vi "mqtt payload to integer.vi"(2 "integer type":i32, 7 "MQTT payload":string="MQTT payload") -> (8 "double":i32, 13 "error out":errorcluster)   [LabVIEW 2017]
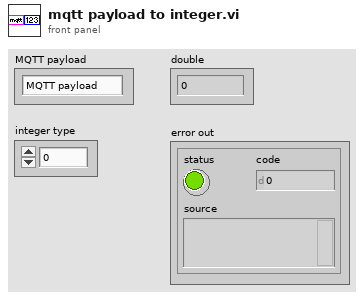
[diagram p1: front panel]
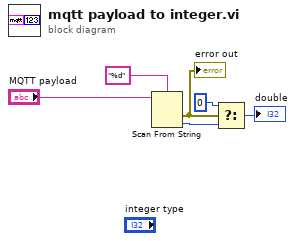
[diagram p0: block diagram]
diagram:
  n1 = Scan From String(format string="%d", input string="MQTT payload") -> (error out=w4:errorcluster, output 1=w2:i32)  [unwired: 3 in, 2 out]
  "error out" <- w4
  n2 = Select(t=0, s=w4, f=w2) -> (s? t:f=→"double":i32)
